vi "Initialize.vi"(8 "error in (no error)":errorcluster, 11 "LogicIO in":refnum<class "LogicIO.lvclass">) -> (0 "error out":errorcluster, 3 "LogicIO out":refnum<class "LogicIO.lvclass">)   [LabVIEW 2016, in "Hardware.lvlib" / "LogicIO.lvlib" / "LogicIO.lvclass"]
uses:
  <userlib>/Common Components/Hardware/LogicIO/LogicIO/LogicIO.lvclass
  <userlib>/Common Components/Hardware/LogicIO/LogicIO/LogicIO.lvclass/LogicIO.ctl
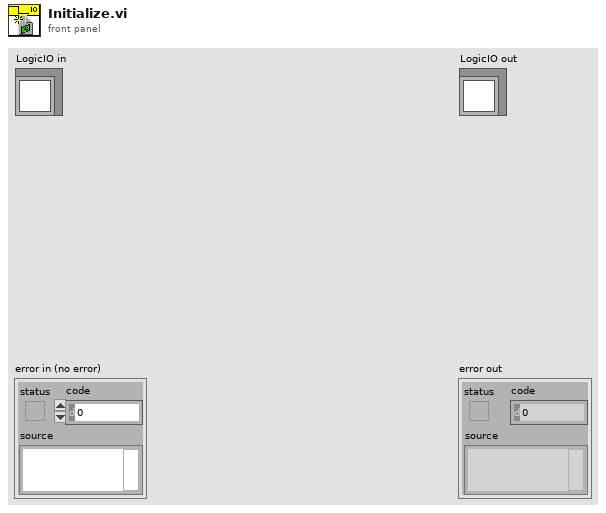
[diagram p1: front panel]
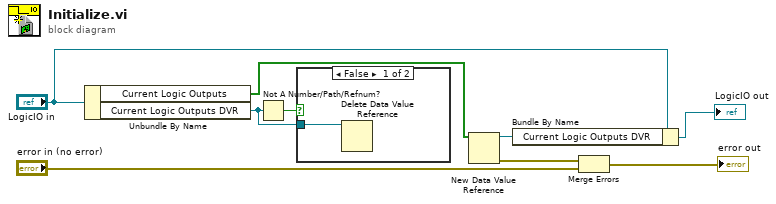
[diagram p0: block diagram]
diagram:
  n1 = Unbundle By Name("LogicIO in") -> ("Current Logic Outputs"=w5:bool[], "Current Logic Outputs DVR"=w4:refnum<data-value>)
  n2 = Not A Number/Path/Refnum?(number/path/refnum=w4) -> (NaN/Path/Refnum?=w3:bool)
  n3 = case shown="False" w3 {
    tunnel: w4 -> [w10 _]
    frame False {
      n4 = Delete Data Value Reference(data value reference=w10) -> ()  [unwired: 1 in, 2 out]
    }
    frame True {
    }
  }
  n5 = New Data Value Reference(data value=w5) -> (data value reference=w7:refnum<data-value>, error out=w8:errorcluster)  [unwired: 1 in]
  n6 = Bundle By Name(cluster="LogicIO in", "Current Logic Outputs DVR"=w7) -> (→"LogicIO out":refnum<class "LogicIO.lvclass">)
  n7 = Merge Errors(w8, "error in (no error)") -> (→"error out":errorcluster)
